vi "getDataFromSQL.vi"(0 "DB":T1, 1 "input_str_PN":string="L0000-110") -> (2 "DateCode8Format_0X30":string, 3 "show_str_labelType":string="None", 4 "show_array_eep":string[][](array[string])=[["11", "11", "0", "0"], ["7", "0", "0", "0"], ["2", "23", "0", "0"], ["0", "80", "0", "0"], ["0", "0", "0", "0"], ["0", "0", "0", "0"], ["0", "0", "0", "0"], ["0", "0", "0", "0"], ["0", "0", "0", "0"], ["0", "80", "0", "0"], ["0", "0", "0", "0"], ["0", "0", "0", "0"], ["0", "FF", "0", "0"], ["0", "0", "0", "0"], ["0", "0", "0", "0"], ["0", "0", "0", "0"], ["0", "0", "0", "0"], ["0", "0", "0", "0"], ["0", "1", "0", "0"], ["0", "A0", "0", "0"], ["0", "4C", "0", "0"], ["0", "55", "0", "0"], ["0", "58", "0", "0"], ["0", "53", "0", "0"], ["0", "48", "0", "0"], ["0", "41", "0", "0"], ["0", "52", "0", "0"], ["0", "45", "0", "0"], ["0", "2D", "0", "0"], ["0", "49", "0", "0"], ["0", "43", "0", "0"], ["0", "54", "0", "0"], ["0", "20", "0", "0"], ["0", "20", "0", "0"], ["0", "20", "0", "0"], ["0", "20", "0", "0"], ["0", "1F", "0", "0"], ["0", "3C", "0", "0"], ["0", "18", "0", "0"], ["0", "A0", "0", "0"], ["0", "48", "0", "0"], ["0", "48", "0", "0"], ["0", "33", "0", "0"], ["0", "43", "0", "0"], ["0", "30", "0", "0"], ["0", "34", "0", "0"], ["0", "30", "0", "0"], ["0", "34", "0", "0"], ["0", "57", "0", "0"], ["0", "34", "0", "0"], ["0", "31", "0", "0"], ["0", "33", "0", "0"], ["0", "57", "0", "0"], ["0", "58", "0", "0"], ["0", "20", "0", "0"], ["0", "20", "0", "0"], ["0", "41", "0", "0"], ["0", "20", "0", "0"], ["0", "3", "0", "0"], ["0", "4", "0", "0"], ["0", "5", "0", "0"], ["0", "8", "0", "0"], ["0", "46", "0", "0"], ["0", "47", "0", "0"], ["0", "B", "0", "0"], ["0", "0", "0", "0"], ["0", "0", "0", "0"], ["0", "0", "0", "0"], ["0", "31", "0", "0"], ["0", "35", "0", "0"], ["0", "32", "0", "0"], ["0", "32", "0", "0"], ["0", "34", "0", "0"], ["0", "34", "0", "0"], ["0", "30", "0", "0"], ["0", "30", "0", "0"], ["0", "35", "0", "0"], ["0", "20", "0", "0"], ["0", "20", "0", "0"], ["0", "20", "0", "0"], ["0", "20", "0", "0"], ["0", "20", "0", "0"], ["0", "20", "0", "0"], ["0", "20", "0", "0"], ["0", "31", "0", "0"], ["0", "35", "0", "0"], ["0", "30", "0", "0"], ["0", "39", "0", "0"], ["0", "30", "0", "0"], ["0", "31", "0", "0"], ["0", "20", "0", "0"], ["0", "20", "0", "0"], ["0", "0", "0", "0"], ["0", "0", "0", "0"], ["0", "67", "0", "0"], ["0", "89", "0", "0"], ["0", "0", "0", "0"], ["0", "0", "0", "0"], ["0", "0", "0", "0"], ["0", "0", "0", "0"], ["0", "0", "0", "0"], ["0", "0", "0", "0"], ["0", "0", "0", "0"], ["0", "0", "0", "0"], ["0", "0", "0", "0"], ["0", "0", "0", "0"], ["0", "0", "0", "0"], ["0", "0", "0", "0"], ["0", "0", "0", "0"], ["0", "0", "0", "0"], ["0", "0", "0", "0"], ["0", "0", "0", "0"], ["0", "0", "0", "0"], ["0", "0", "0", "0"], ["0", "0", "0", "0"], ["0", "0", "0", "0"], ["0", "0", "0", "0"], ["0", "0", "0", "0"], ["0", "0", "0", "0"], ["0", "0", "0", "0"], ["0", "0", "0", "0"], ["0", "0", "0", "0"], ["0", "0", "0", "0"], ["0", "0", "0", "0"], ["0", "0", "0", "0"], ["0", "0", "0", "0"], ["0", "0", "0", "0"], ["0", "0", "0", "0"]], 5 "show_str_createDate":string, 6 "show_bool_valid":bool=TRUE, 7 "show_bool_exsit":bool=TRUE, 8 "show_str_message":string="该PN对应的文件属于SWR！\n有效日期段为：\n2015/11/16 8:14:18,2015/11/23 8:14:18", 9 "PN description":string)   [LabVIEW 2011]
uses:
  <vilib>/Utility/file.llb/Read From Spreadsheet File (string).vi
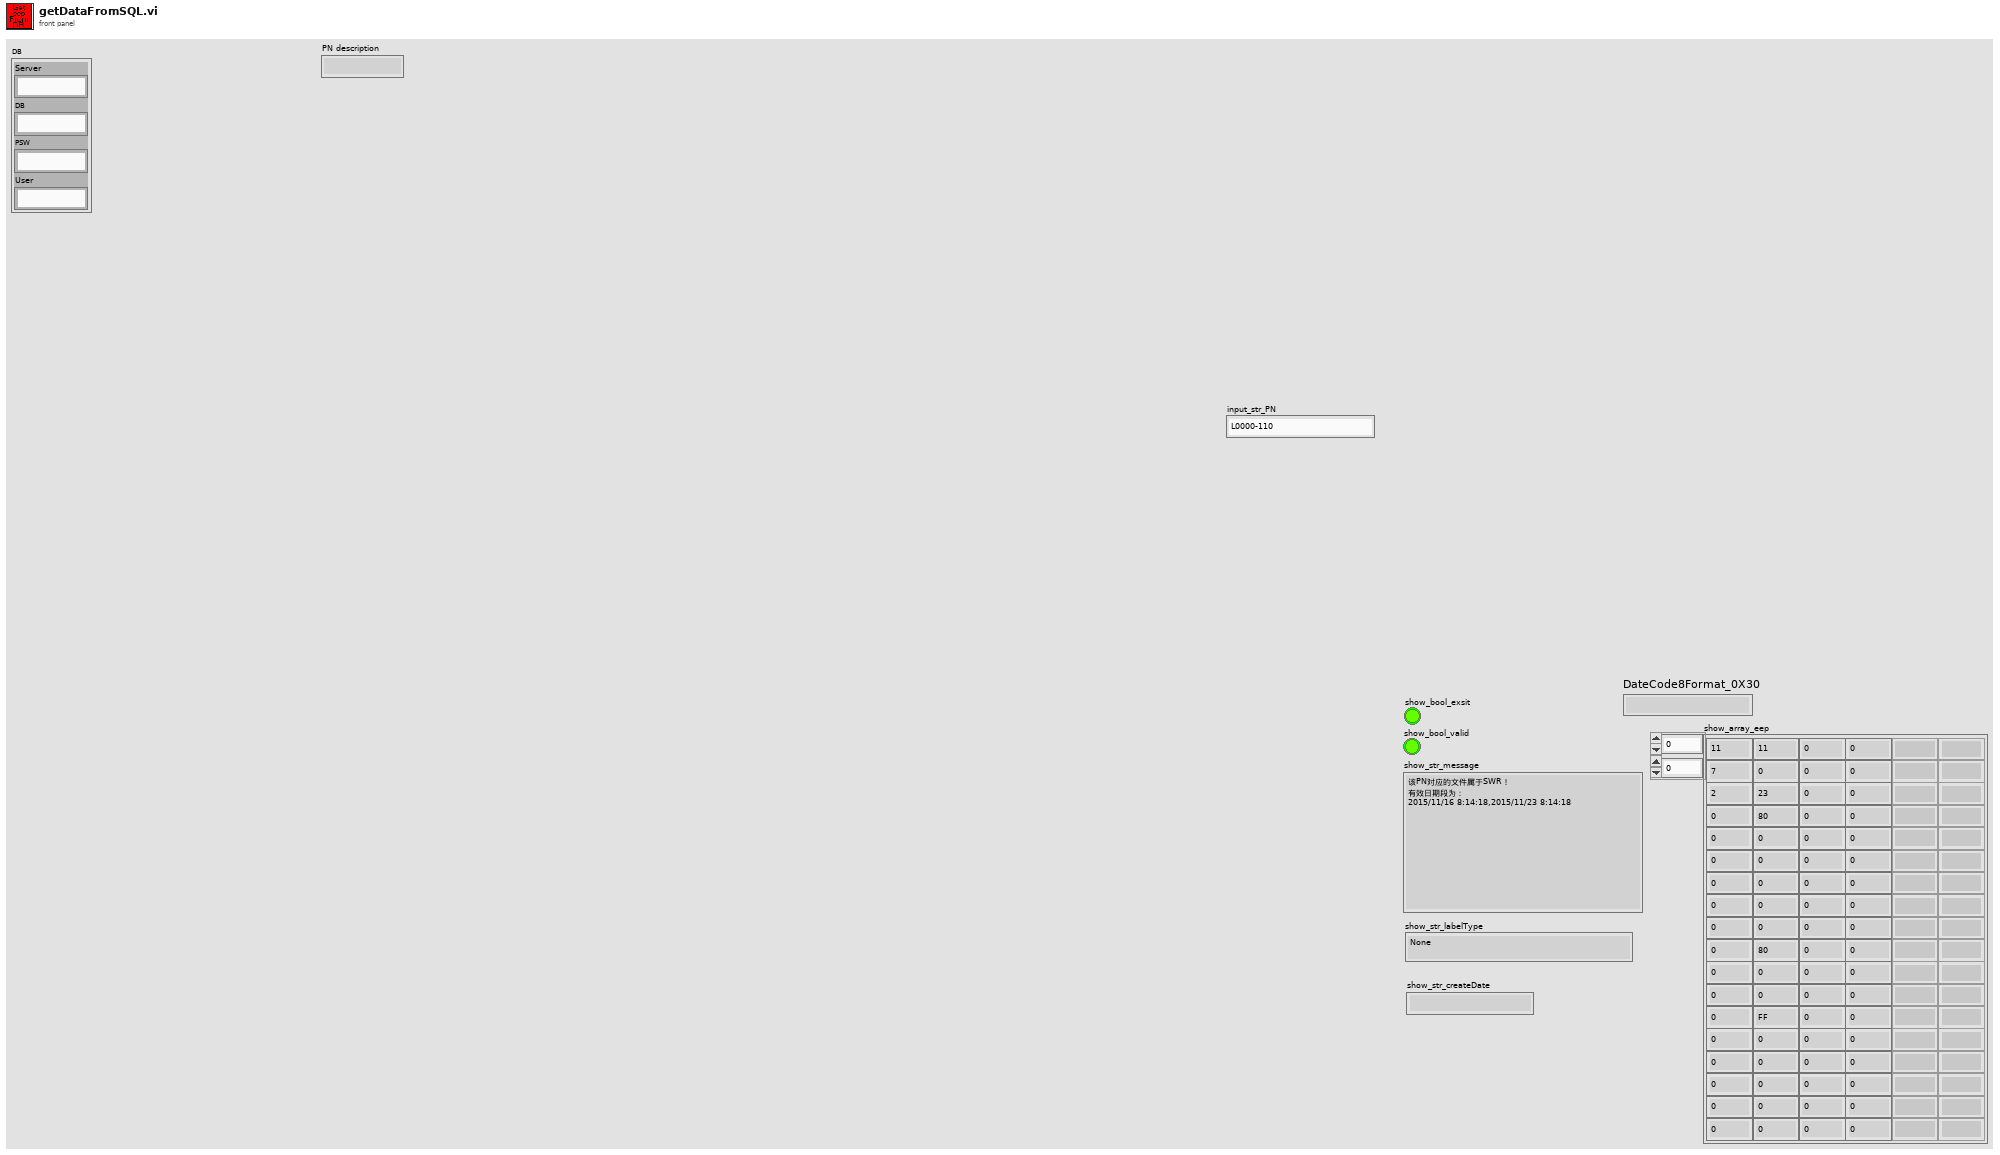
[diagram p1: front panel]
types:
  T1 = cluster{"Server":string, "DB":string, "PSW":string, "User":string}
  T2 = enum16{"查询表名", "查询列名", "查询记录", "查询总记录", "查询数据", "转换数据"}
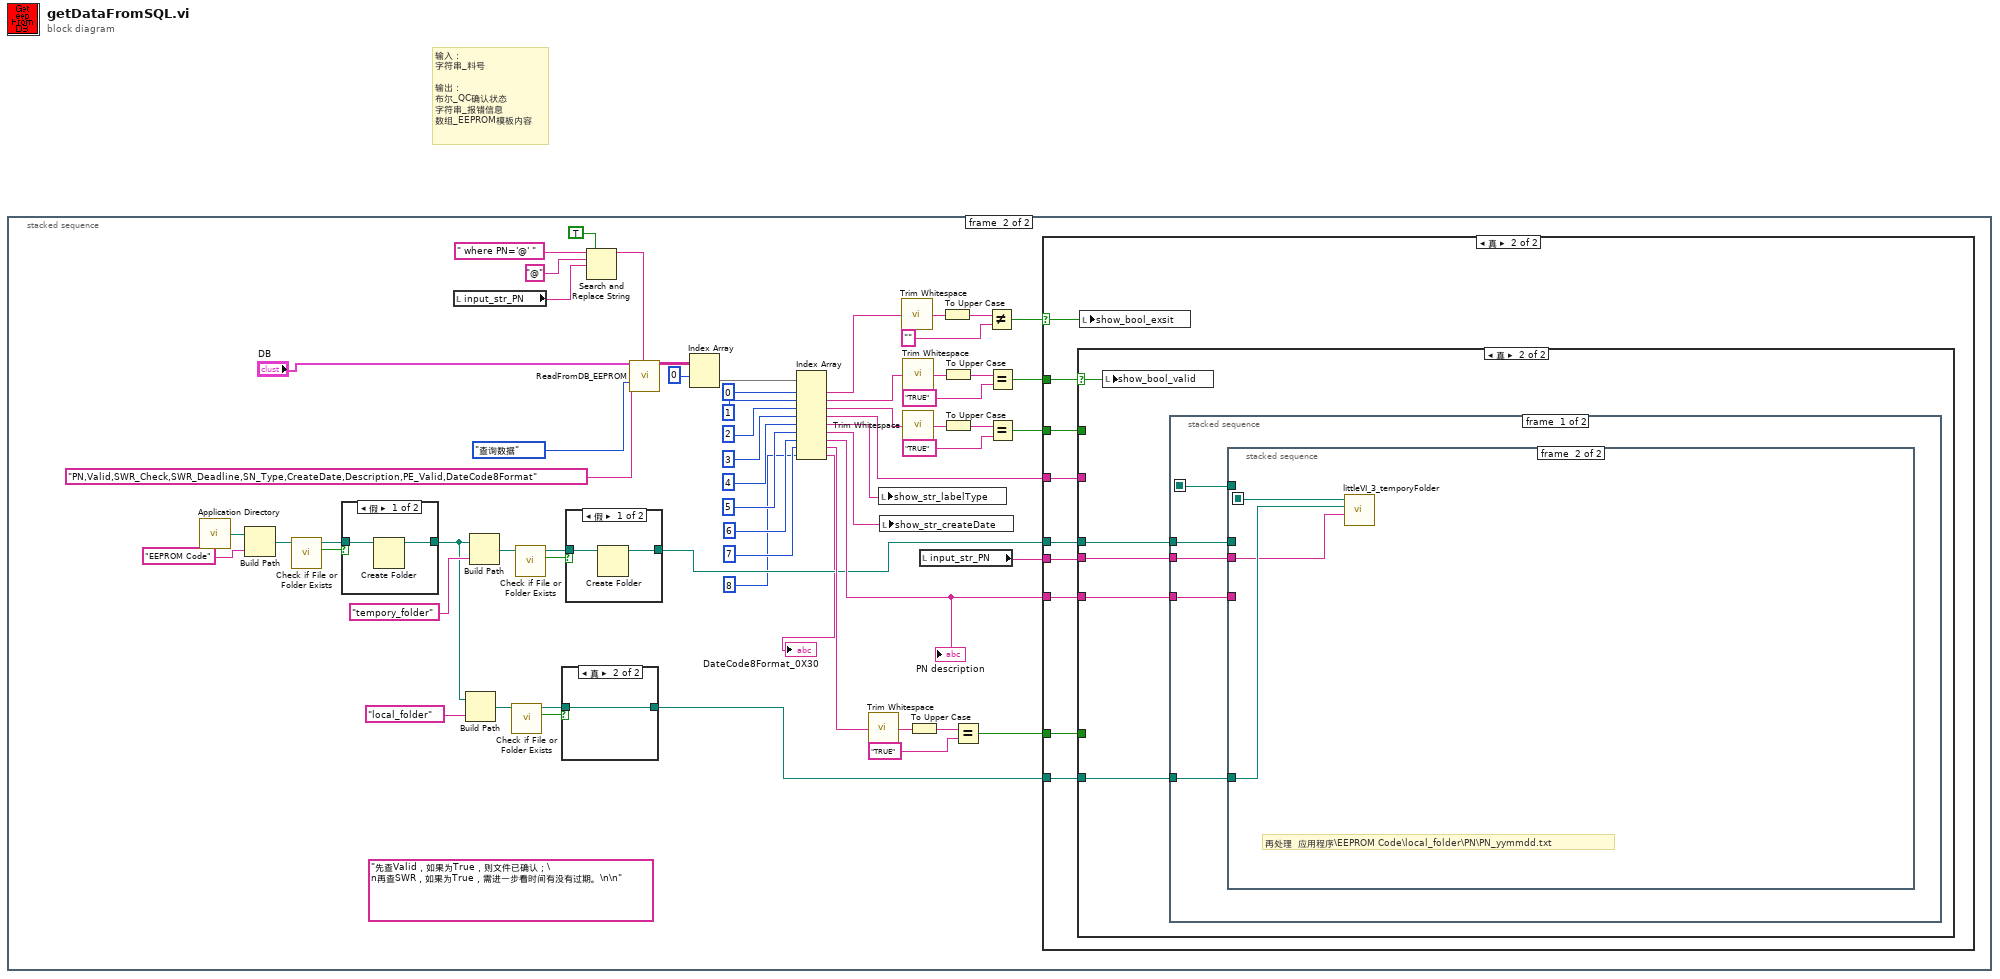
[diagram p0: block diagram]
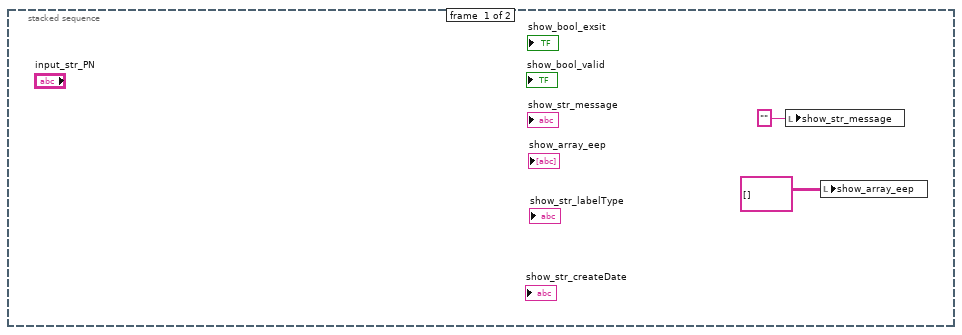
[diagram p2: hidden frame]
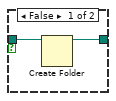
[diagram p3: hidden frame]
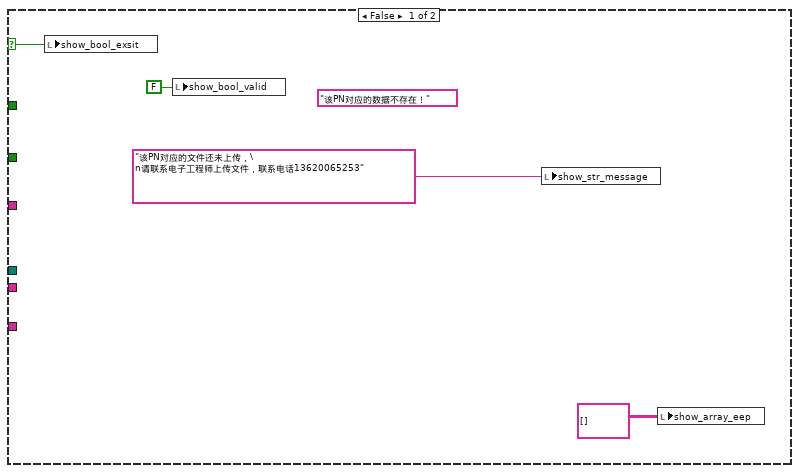
[diagram p5: hidden frame]
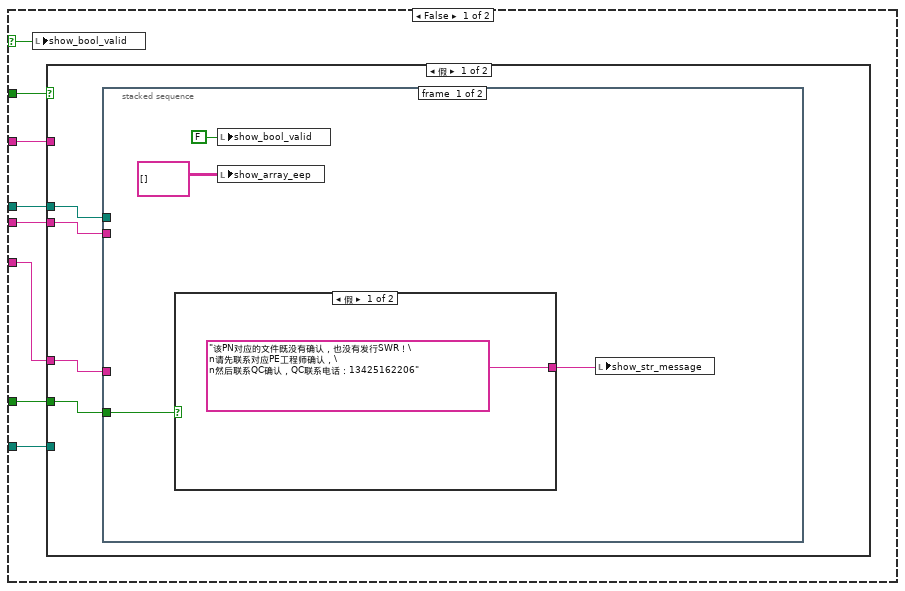
[diagram p6: hidden frame]
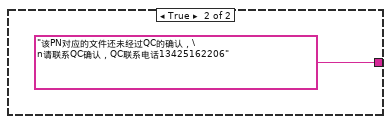
[diagram p7: hidden frame]
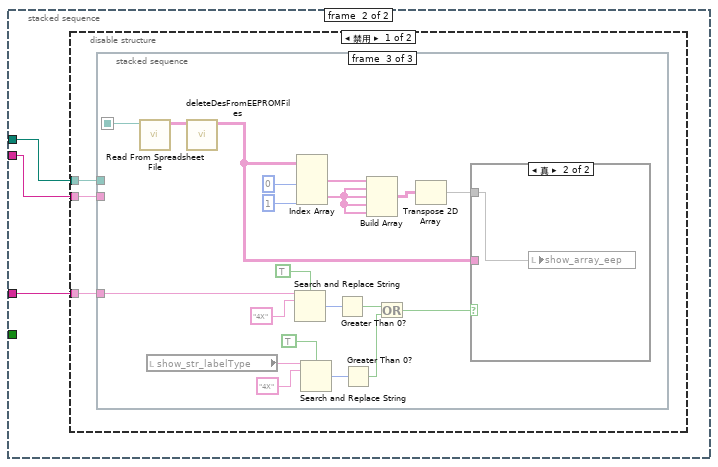
[diagram p8: hidden frame]
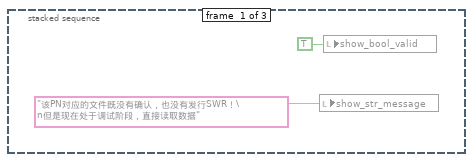
[diagram p9: hidden frame]
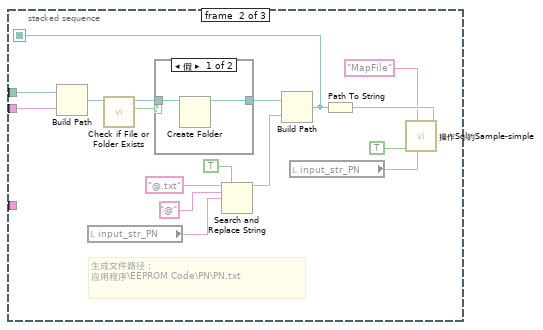
[diagram p10: hidden frame]
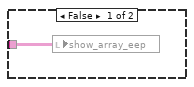
[diagram p12: hidden frame]
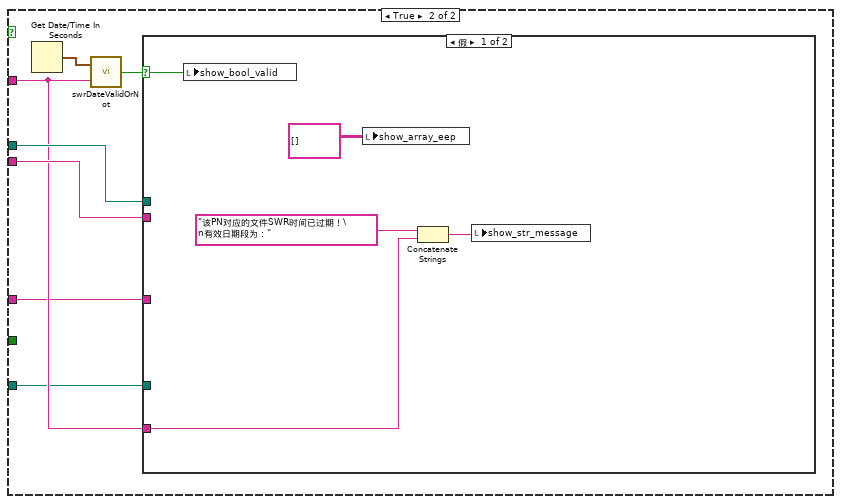
[diagram p14: hidden frame]
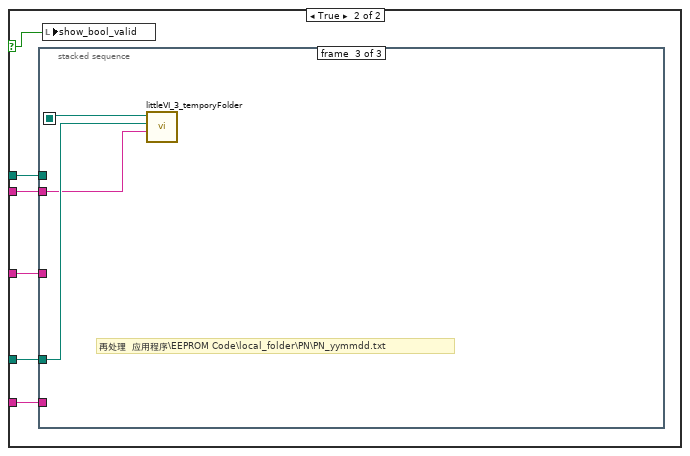
[diagram p15: hidden frame]
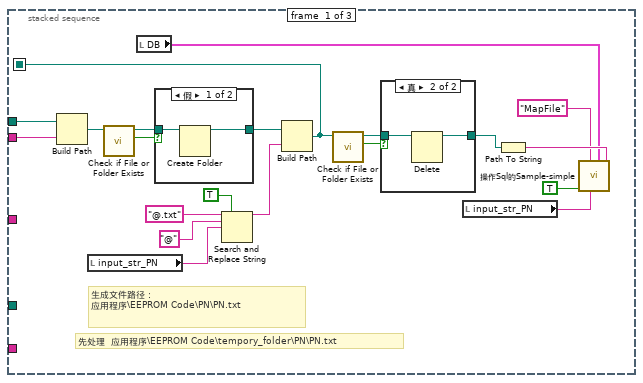
[diagram p16: hidden frame]
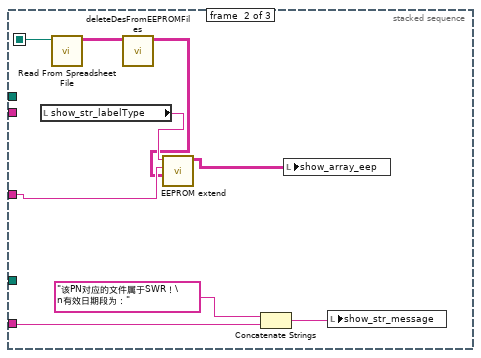
[diagram p19: hidden frame]
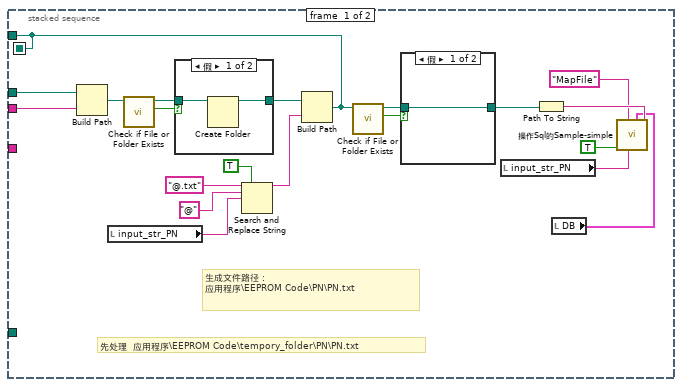
[diagram p20: hidden frame]
diagram:
  # "输入：\n字符串_料号\n\n输出：\n布尔_QC确认状态\n字符串_报错信息\n数组_EEPROM模板内容"
  n1 = stacked-sequence {
    frame #0 {
      n2 = local write "show_str_message"("" ("show_str_message")) -> ()
      n3 = local write "show_array_eep"(string[][] [] ("show_array_eep")) -> ()
    }
    frame #1 {
      (unwired) "先查Valid，如果为True，则文件已确认；\n再查SWR，如果为True，需进一步看时间有没有过期。\n\n"
      n4 = call <vilib>:"Application Directory.vi"() -> ("Application Directory"=w50:path)
      n5 = Build Path(base path=w50, name or relative path="EEPROM Code" ("名称或相对路径")) -> (appended path=w52:path)
      n6 = call <vilib>:"Check if File or Folder Exists.vi"("path"=w52) -> ("file or folder exists?"=w53:bool, "dup path"=w54:path)  [unwired: 8 in, 1 out]
      n7 = case shown="假" w53 {
        tunnel: w54 -> [w258 w259]
        tunnel: [w257 w259] -> w8
        frame False {
          n8 = Create Folder(path (use dialog)=w258) -> (created path=w257:path)  [unwired: 2 in, 2 out]
        }
        frame True {
        }
      }
      n9 = local read "input_str_PN"() -> (w49:string)
      n10 = Build Path(base path=w8, name or relative path="local_folder" ("名称或相对路径")) -> (appended path=w9:path)
      n11 = Build Path(base path=w8, name or relative path="tempory_folder" ("名称或相对路径")) -> (appended path=w16:path)
      n12 = call <vilib>:"Check if File or Folder Exists.vi"("path"=w9) -> ("file or folder exists?"=w10:bool, "dup path"=w11:path)  [unwired: 8 in, 1 out]
      n13 = call <vilib>:"Check if File or Folder Exists.vi"("path"=w16) -> ("file or folder exists?"=w15:bool, "dup path"=w14:path)  [unwired: 8 in, 1 out]
      n14 = case shown="真" w10 {
        tunnel: w11 -> [w66 w67]
        tunnel: [w65 w67] -> w6
        frame False {
          n15 = Create Folder(path (use dialog)=w66) -> (created path=w65:path)  [unwired: 2 in, 2 out]
        }
        frame True {
        }
      }
      n16 = case shown="假" w15 {
        tunnel: w14 -> [w69 w70]
        tunnel: [w68 w70] -> w12
        frame False {
          n17 = Create Folder(path (use dialog)=w69) -> (created path=w68:path)  [unwired: 2 in, 2 out]
        }
        frame True {
        }
      }
      n18 = Search and Replace String(replace all?=TRUE ("替换全部？(F)"), input string=" where PN='@' ", search string="@" ("搜索字符串"), replace string=w49) -> (result string=w59:string)  [unwired: 4 in, 3 out]
      n19 = call "ReadFromDB_EEPROM.vi"("DB"="DB", "操作模式"=T2."查询数据", "查询项目"="PN,Valid,SWR_Check,SWR_Deadline,SN_Type,CreateDate,Description,PE_Valid,DateCode8Format", "限定条件"=w59) -> ("ConvertToArray"=w47:string[][])  [unwired: 13 in, 10 out]
      n20 = Index Array(array=w47, index (row)=0 ("索引 (行)")) -> (element=w45:string[])  [unwired: 1 in]
      n21 = Index Array(array=w45, index #1=0 ("索引"), index #2=1 ("索引"), index #3=2 ("索引"), index #4=3 ("索引"), index #5=4 ("索引"), index #6=5 ("索引"), index #7=6 ("索引"), index #8=7 ("索引"), index #9=8 ("索引")) -> (element #1=w39:string, element #2=w38:string, element #3=w32:string, element #4=w28:string, element #5=w27:string, element #6=w26:string, element #7=w23:string, element #8=w18:string, element #9=→"DateCode8Format_0X30":string)
      "PN description" <- w23
      n22 = call <vilib>:"Trim Whitespace.vi"("string"=w18) -> ("trimmed string"=w21:string)  [unwired: 1 in]
      n23 = local write "show_str_labelType"(w27) -> ()
      n24 = local write "show_str_createDate"(w26) -> ()
      n25 = call <vilib>:"Trim Whitespace.vi"("string"=w39) -> ("trimmed string"=w40:string)  [unwired: 1 in]
      n26 = call <vilib>:"Trim Whitespace.vi"("string"=w38) -> ("trimmed string"=w58:string)  [unwired: 1 in]
      n27 = call <vilib>:"Trim Whitespace.vi"("string"=w32) -> ("trimmed string"=w33:string)  [unwired: 1 in]
      n28 = To Upper Case(1:w21) -> (0:w20:string)
      n29 = local read "input_str_PN"() -> (w48:string)
      n30 = To Upper Case(1:w40) -> (0:w41:string)
      n31 = To Upper Case(1:w58) -> (0:w57:string)
      n32 = To Upper Case(1:w33) -> (0:w34:string)
      n33 = Equal?(x=w20, y="TRUE") -> (x = y?=w17:bool)
      n34 = Not Equal?(x=w41, y="") -> (x != y?=w37:bool)
      n35 = Equal?(x=w57, y="TRUE") -> (x = y?=w55:bool)
      n36 = Equal?(x=w34, y="TRUE") -> (x = y?=w31:bool)
      n37 = case shown="真" w37 {
        selector: w37 -> [w74 w80]
        tunnel: w55 -> [_ w83]
        tunnel: w12 -> [_ w82]
        tunnel: w48 -> [_ w81]
        tunnel: w31 -> [_ w79]
        tunnel: w28 -> [_ w78]
        tunnel: w23 -> [_ w77]
        tunnel: w17 -> [_ w76]
        tunnel: w6 -> [_ w75]
        frame False {
          (unwired) "该PN对应的数据不存在！"
          n38 = local write "show_bool_exsit"(w74) -> ()
          n39 = local write "show_bool_valid"(FALSE ("show_bool_valid")) -> ()
          n40 = local write "show_str_message"("该PN对应的文件还未上传，\n请联系电子工程师上传文件，联系电话13620065253") -> ()
          n41 = local write "show_array_eep"(string[][] [] ("show_array_eep")) -> ()
        }
        frame True {
          n42 = case shown="真" w83 {
            selector: w83 -> [w91 w211]
            tunnel: w82 -> [w88 w210]
            tunnel: w81 -> [w87 w209]
            tunnel: w79 -> [w90 _]
            tunnel: w78 -> [w89 _]
            tunnel: w77 -> [w86 w208]
            tunnel: w76 -> [w85 _]
            tunnel: w75 -> [w84 w207]
            frame False {
              n43 = local write "show_bool_valid"(w91) -> ()
              n44 = case shown="假" w90 {
                tunnel: w89 -> [_ w153]
                tunnel: w88 -> [w95 w155]
                tunnel: w87 -> [w94 w154]
                tunnel: w86 -> [w93 w152]
                tunnel: w85 -> [w92 _]
                tunnel: w84 -> [_ w151]
                frame False {
                  n45 = stacked-sequence {
                    tunnel: w95 -> [_ w104]
                    tunnel: w94 -> [_ w103]
                    tunnel: w93 -> [_ w102]
                    tunnel: w92 -> [w97 _]
                    frame #0 {
                      n46 = case shown="假" w97 {
                        tunnel: ["该PN对应的文件既没有确认，也没有发行SWR！\n请先联系对应PE工程师确认，\n然后联系QC确认，QC联系电话：13425162206" "该PN对应的文件还未经过QC的确认，\n请联系QC确认，QC联系电话13425162206"] -> w96
                        frame False {
                        }
                        frame True {
                        }
                      }
                      n47 = local write "show_bool_valid"(FALSE ("show_bool_valid")) -> ()
                      n48 = local write "show_array_eep"(string[][] [] ("show_array_eep")) -> ()
                      n49 = local write "show_str_message"(w96) -> ()
                    }
                    frame #1 {
                      n50 = disable-structure shown="禁用" {
                        disable-tunnel: w104 -> [w107 _]
                        disable-tunnel: w103 -> [w106 _]
                        disable-tunnel: w102 -> [w105 _]
                        frame Disabled {
                          n51 = stacked-sequence {
                            seq-local: [_ w111 _] -> [_ _ w148]
                            tunnel: w107 -> [_ w120 _]
                            tunnel: w106 -> [_ w119 _]
                            tunnel: w105 -> [_ _ w136]
                            frame #0 {
                              n52 = local write "show_str_message"("该PN对应的文件既没有确认，也没有发行SWR！\n但是现在处于调试阶段，直接读取数据") -> ()
                              n53 = local write "show_bool_valid"(TRUE ("show_bool_valid")) -> ()
                            }
                            frame #1 {
                              # "生成文件路径：\n应用程序\\EEPROM Code\\PN\\PN.txt"
                              n54 = Build Path(base path=w120, name or relative path=w119) -> (appended path=w123:path)
                              n55 = local read "input_str_PN"() -> (w115:string)
                              n56 = call <vilib>:"Check if File or Folder Exists.vi"("path"=w123) -> ("file or folder exists?"=w122:bool, "dup path"=w121:path)  [unwired: 8 in, 1 out]
                              n57 = case shown="假" w122 {
                                tunnel: w121 -> [w127 w128]
                                tunnel: [w126 w128] -> w114
                                frame False {
                                n58 = Create Folder(path (use dialog)=w127) -> (created path=w126:path)  [unwired: 2 in, 2 out]
                                }
                                frame True {
                                }
                              }
                              n59 = Search and Replace String(replace all?=TRUE ("替换全部？(F)"), input string="@.txt", search string="@" ("搜索字符串"), replace string=w115) -> (result string=w113:string)  [unwired: 4 in, 3 out]
                              n60 = Build Path(base path=w114, name or relative path=w113) -> (appended path=w111:path)
                              n61 = local read "input_str_PN"() -> (w124:string)
                              n62 = Path To String(path=w111) -> (string=w112:string)
                              n63 = call "操作Sql的Sample-simple.vi"("SavefileName"=w112, "sn 2"=w124, "fieldName"="MapFile", "下载文件"=TRUE) -> ()  [unwired: 8 in]
                            }
                            frame #2 {
                              n64 = call-poly <vilib>:"Read From Spreadsheet File.vi"("file path (dialog if empty)"=w148) -> ("all rows"=w130:string[][])  [unwired: 6 in, 4 out]
                              n65 = local read "show_str_labelType"() -> (w147:string)
                              n66 = call "deleteDesFromEEPROMFiles.vi"("input_eeprom"=w130) -> ("show_eeprom"=w129:string[][])  [unwired: 10 in]
                              n67 = Search and Replace String(case sensitive?=TRUE ("忽略大小写？(F)"), input string=w136, search string="4X" ("搜索字符串")) -> (number of replacements=w139:i32)  [unwired: 5 in, 3 out]
                              n68 = Index Array(array=w129, index (col) #1=0 ("禁用的索引 (列)"), index (col) #2=1 ("索引 (列)")) -> (element #1=w141:string[], element #2=w131:string[])  [unwired: 2 in]
                              n69 = Search and Replace String(case sensitive?=TRUE ("忽略大小写？(F)"), input string=w147, search string="4X" ("搜索字符串")) -> (number of replacements=w144:i32)  [unwired: 5 in, 3 out]
                              n70 = Greater Than 0?(x=w139) -> (x > 0?=w135:bool)
                              n71 = Greater Than 0?(x=w144) -> (x > 0?=w134:bool)
                              n72 = Build Array(w141, w131, w131, w131, w131) -> (w140:string[][])
                              n73 = Or(x=w135, y=w134) -> (x .or. y?=w133:bool)
                              n74 = Transpose 2D Array(2D array=w140) -> (transposed array=w132:string[][])
                              n75 = case shown="真" w133 {
                                tunnel: w129 -> [w149 _]
                                tunnel: w132 -> [_ w150]
                                frame False {
                                n76 = local write "show_array_eep"(w149) -> ()
                                }
                                frame True {
                                n77 = local write "show_array_eep"(w150) -> ()
                                }
                              }
                            }
                          }
                        }
                        frame Enabled {
                        }
                      }
                    }
                  }
                }
                frame True {
                  n78 = Get Date/Time In Seconds() -> (seconds since 1Jan1904=w157:timestamp)
                  n79 = call "swrDateValidOrNot.vi"("input_date_start&endDate"=w153, "input_date_system"=w157) -> ("show_dateInRange"=w156:bool)
                  n80 = case shown="假" w156 {
                    selector: w156 -> [w158 w165]
                    tunnel: w155 -> [_ w168]
                    tunnel: w154 -> [_ w167]
                    tunnel: w153 -> [w160 w166]
                    tunnel: w152 -> [_ w164]
                    tunnel: w151 -> [_ w163]
                    frame False {
                      n81 = local write "show_bool_valid"(w158) -> ()
                      n82 = local write "show_array_eep"(string[][] [] ("show_array_eep")) -> ()
                      n83 = Concatenate Strings("该PN对应的文件SWR时间已过期！\n有效日期段为：", w160) -> (w159:string)
                      n84 = local write "show_str_message"(w159) -> ()
                    }
                    frame True {
                      n85 = stacked-sequence {
                        seq-local: [w171 _ _] -> [_ w203 w206]
                        tunnel: w168 -> [w183 _ _]
                        tunnel: w167 -> [w182 _ w204]
                        tunnel: w166 -> [_ w201 _]
                        tunnel: w164 -> [_ w197 _]
                        tunnel: w163 -> [_ _ w205]
                        frame #0 {
                          # "先处理  应用程序\\EEPROM Code\\tempory_folder\\PN\\PN.txt"
                          # "生成文件路径：\n应用程序\\EEPROM Code\\PN\\PN.txt"
                          n86 = Build Path(base path=w183, name or relative path=w182) -> (appended path=w186:path)
                          n87 = local read "input_str_PN"() -> (w178:string)
                          n88 = call <vilib>:"Check if File or Folder Exists.vi"("path"=w186) -> ("file or folder exists?"=w185:bool, "dup path"=w184:path)  [unwired: 8 in, 1 out]
                          n89 = local read "DB"() -> (w169:T1)
                          n90 = case shown="假" w185 {
                            tunnel: w184 -> [w193 w194]
                            tunnel: [w192 w194] -> w177
                            frame False {
                              n91 = Create Folder(path (use dialog)=w193) -> (created path=w192:path)  [unwired: 2 in, 2 out]
                            }
                            frame True {
                            }
                          }
                          n92 = Search and Replace String(replace all?=TRUE ("替换全部？(F)"), input string="@.txt", search string="@" ("搜索字符串"), replace string=w178) -> (result string=w176:string)  [unwired: 4 in, 3 out]
                          n93 = Build Path(base path=w177, name or relative path=w176) -> (appended path=w171:path)
                          n94 = call <vilib>:"Check if File or Folder Exists.vi"("path"=w171) -> ("file or folder exists?"=w173:bool, "dup path"=w172:path)  [unwired: 8 in, 1 out]
                          n95 = case shown="真" w173 {
                            tunnel: w172 -> [w189 w191]
                            tunnel: [w189 w190] -> w170
                            frame False {
                            }
                            frame True {
                              n96 = Delete(path (use dialog)=w191) -> (deleted path=w190:path)  [unwired: 4 in, 2 out]
                            }
                          }
                          n97 = local read "input_str_PN"() -> (w187:string)
                          n98 = Path To String(path=w170) -> (string=w175:string)
                          n99 = call "操作Sql的Sample-simple.vi"("SavefileName"=w175, "DB"=w169, "sn 2"=w187, "fieldName"="MapFile", "下载文件"=TRUE) -> ()  [unwired: 7 in]
                        }
                        frame #1 {
                          n100 = local read "show_str_labelType"() -> (w198:string)
                          n101 = call-poly <vilib>:"Read From Spreadsheet File.vi"("file path (dialog if empty)"=w203) -> ("all rows"=w199:string[][])  [unwired: 6 in, 4 out]
                          n102 = call "deleteDesFromEEPROMFiles.vi"("input_eeprom"=w199) -> ("show_eeprom"=w196:string[][])  [unwired: 10 in]
                          n103 = call "EEPROM extend.vi"("input_eeprom"=w196, "lableDescription"=w197, "lableType"=w198) -> ("out_put_eeprom"=w195:string[][])  [unwired: 8 in]
                          n104 = Concatenate Strings("该PN对应的文件属于SWR！\n有效日期段为：", w201) -> (w200:string)
                          n105 = local write "show_array_eep"(w195) -> ()
                          n106 = local write "show_str_message"(w200) -> ()
                        }
                        frame #2 {
                          # "再处理  应用程序\\EEPROM Code\\local_folder\\PN\\PN_yymmdd.txt"
                          n107 = call "littleVI_3_temporyFolder.vi"("input_PN"=w204, "EEPROM一级目录"=w205, "文件路径"=w206) -> ()  [unwired: 9 in]
                        }
                      }
                      n108 = local write "show_bool_valid"(w165) -> ()
                    }
                  }
                }
              }
            }
            frame True {
              n109 = local write "show_bool_valid"(w211) -> ()
              n110 = stacked-sequence {
                seq-local: [w215 _] -> [_ w256]
                tunnel: w210 -> [w214 _]
                tunnel: w209 -> [w216 _]
                tunnel: w208 -> [w213 w249]
                tunnel: w207 -> [w212 _]
                frame #0 {
                  n111 = stacked-sequence {
                    seq-local: [w218 _] -> [_ w245]
                    tunnel: w216 -> [w231 w243]
                    tunnel: [w218 _] -> w215
                    tunnel: w214 -> [w219 _]
                    tunnel: w213 -> [_ _]
                    tunnel: w212 -> [_ w244]
                    frame #0 {
                      # "先处理  应用程序\\EEPROM Code\\tempory_folder\\PN\\PN.txt"
                      # "生成文件路径：\n应用程序\\EEPROM Code\\PN\\PN.txt"
                      n112 = Build Path(base path=w219, name or relative path=w231) -> (appended path=w234:path)
                      n113 = local read "input_str_PN"() -> (w227:string)
                      n114 = call <vilib>:"Check if File or Folder Exists.vi"("path"=w234) -> ("file or folder exists?"=w233:bool, "dup path"=w232:path)  [unwired: 8 in, 1 out]
                      n115 = case shown="假" w233 {
                        tunnel: w232 -> [w241 w242]
                        tunnel: [w240 w242] -> w226
                        frame False {
                          n116 = Create Folder(path (use dialog)=w241) -> (created path=w240:path)  [unwired: 2 in, 2 out]
                        }
                        frame True {
                        }
                      }
                      n117 = Search and Replace String(replace all?=TRUE ("替换全部？(F)"), input string="@.txt", search string="@" ("搜索字符串"), replace string=w227) -> (result string=w225:string)  [unwired: 4 in, 3 out]
                      n118 = Build Path(base path=w226, name or relative path=w225) -> (appended path=w218:path)
                      n119 = call <vilib>:"Check if File or Folder Exists.vi"("path"=w218) -> ("file or folder exists?"=w222:bool, "dup path"=w221:path)  [unwired: 8 in, 1 out]
                      n120 = case shown="假" w222 {
                        tunnel: w221 -> [w237 w239]
                        tunnel: [w237 w238] -> w220
                        frame False {
                        }
                        frame True {
                          n121 = Delete(path (use dialog)=w239) -> (deleted path=w238:path)  [unwired: 4 in, 2 out]
                        }
                      }
                      n122 = local read "input_str_PN"() -> (w235:string)
                      n123 = Path To String(path=w220) -> (string=w224:string)
                      n124 = local read "DB"() -> (w217:T1)
                      n125 = call "操作Sql的Sample-simple.vi"("SavefileName"=w224, "DB"=w217, "sn 2"=w235, "fieldName"="MapFile", "下载文件"=TRUE) -> ()  [unwired: 7 in]
                    }
                    frame #1 {
                      # "再处理  应用程序\\EEPROM Code\\local_folder\\PN\\PN_yymmdd.txt"
                      n126 = call "littleVI_3_temporyFolder.vi"("input_PN"=w243, "EEPROM一级目录"=w244, "文件路径"=w245) -> ()  [unwired: 9 in]
                    }
                  }
                }
                frame #1 {
                  n127 = call-poly <vilib>:"Read From Spreadsheet File.vi"("file path (dialog if empty)"=w256) -> ("all rows"=w250:string[][])  [unwired: 6 in, 4 out]
                  n128 = call "deleteDesFromEEPROMFiles.vi"("input_eeprom"=w250) -> ("show_eeprom"=w247:string[][])  [unwired: 10 in]
                  n129 = local read "show_str_labelType"() -> (w246:string)
                  n130 = local read "show_str_createDate"() -> (w252:string)
                  n131 = local read "show_str_labelType"() -> (w255:string)
                  n132 = call "EEPROM extend.vi"("input_eeprom"=w247, "lableDescription"=w249, "lableType"=w246) -> ("out_put_eeprom"=w248:string[][])  [unwired: 8 in]
                  n133 = Concatenate Strings(w255, "\n", "Create Date：", w252) -> (w251:string)
                  n134 = local write "show_array_eep"(w248) -> ()
                  n135 = local write "show_str_message"(w251) -> ()
                }
              }
            }
          }
          n136 = local write "show_bool_exsit"(w80) -> ()
        }
      }
    }
  }
